vi "calc_deltaF_x2.vi"(8 "valid in":bool, 11 "Data in":fxp<+/-,16,14>[](array[numeric])=[0.0, 0.0, 0.0, 0.0]) -> (0 "valid out":bool, 2 "deltaF":fxp<+/-,32,30>[](array[numeric]), 3 "Data out":fxp<+/-,16,14>[](array[numeric]))   [LabVIEW 2013]
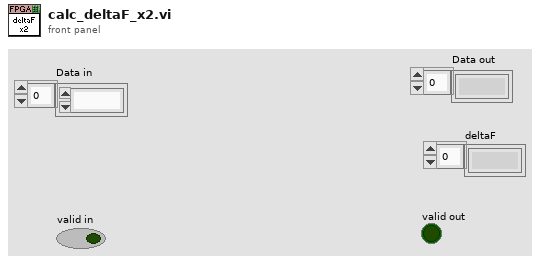
[diagram p1: front panel]
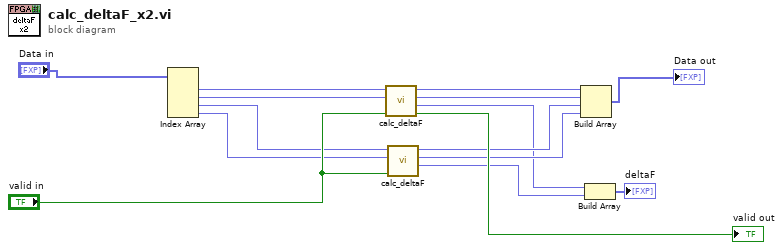
[diagram p0: block diagram]
diagram:
  n1 = Index Array(array="Data in") -> (element #1=w14:fxp<+/-,16,14>, element #2=w13:fxp<+/-,16,14>, element #3=w7:fxp<+/-,16,14>, element #4=w6:fxp<+/-,16,14>)  [unwired: 4 in]
  n2 = call "calc_deltaF.vi"("valid in"="valid in", "Q in"=w13, "I in"=w14) -> ("output valid"=→"valid out":bool, "delta_F"=w3:fxp<+/-,32,30>, "Q out"=w11:fxp<+/-,16,14>, "I out"=w12:fxp<+/-,16,14>)  [unwired: 5 in]
  n3 = call "calc_deltaF.vi"("valid in"="valid in", "Q in"=w6, "I in"=w7) -> ("delta_F"=w2:fxp<+/-,32,30>, "Q out"=w4:fxp<+/-,16,14>, "I out"=w5:fxp<+/-,16,14>)  [unwired: 5 in, 1 out]
  n4 = Build Array(w12, w11, w5, w4) -> (→"Data out":fxp<+/-,16,14>[])
  n5 = Build Array(w3, w2) -> (→"deltaF":fxp<+/-,32,30>[])
